vi "DCMotor.vi"(0 "V":dbl, 5 "Omega":dbl, 7 "I":dbl, 9 "dt":dbl, 11 "error in (no error)":errorcluster) -> (4 "Omega Out":dbl, 6 "I Out":dbl, 10 "Torque Out":dbl, 15 "error out":errorcluster)   [LabVIEW 2017]
uses:
  <vilib>/ptbypt/NI_PtbyPt.lvlib
panel:
  in  "Ng":dbl=8.0
  in  "Cs":dbl=0.03
  in  "Cv":dbl=4e-05
  in  "J":dbl=4e-05
  in  "L":dbl=0.8
  in  "R":dbl=7.0
  in  "K":dbl=0.063
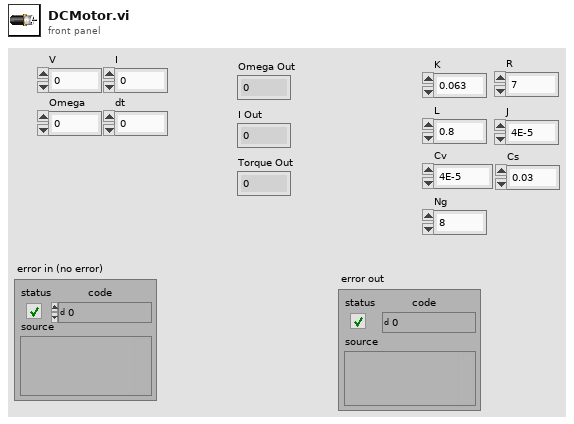
[diagram p1: front panel]
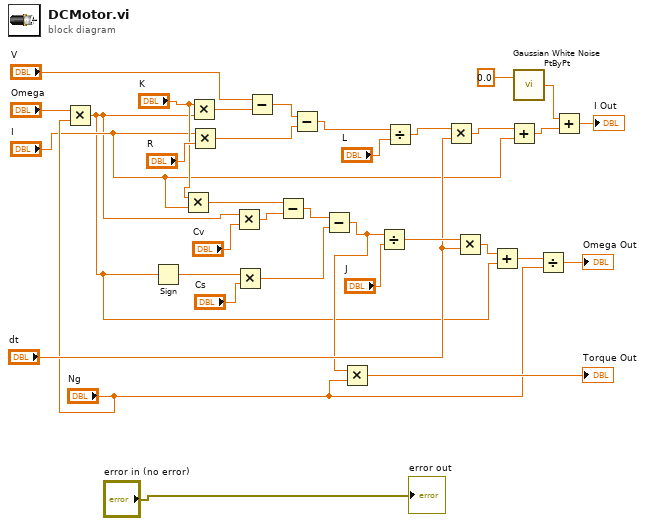
[diagram p0: block diagram]
diagram:
  n1 = Multiply(x="Omega", y="Ng") -> (x*y=w2:dbl)
  n2 = Sign(1:w2) -> (0:w22:dbl)
  n3 = Multiply(x="K", y="I") -> (x*y=w24:dbl)
  n4 = Multiply(x="K", y=w2) -> (x*y=w33:dbl)
  n5 = Multiply(x="I", y="R") -> (x*y=w31:dbl)
  n6 = Multiply(x=w2, y="Cv") -> (x*y=w23:dbl)
  n7 = Multiply(x=w22, y="Cs") -> (x*y=w19:dbl)
  n8 = Subtract(x="V", y=w33) -> (x-y=w32:dbl)
  n9 = Subtract(x=w24, y=w23) -> (x-y=w20:dbl)
  n10 = Subtract(x=w32, y=w31) -> (x-y=w29:dbl)
  n11 = Subtract(x=w20, y=w19) -> (x-y=w14:dbl)
  n12 = Multiply(x=w14, y="Ng") -> (x*y=→"Torque Out":dbl)
  n13 = Divide(x=w14, y="J") -> (x/y=w17:dbl)
  n14 = Divide(x=w29, y="L") -> (x/y=w28:dbl)
  n15 = Multiply(x=w28, y="dt") -> (x*y=w27:dbl)
  n16 = Multiply(x=w17, y="dt") -> (x*y=w15:dbl)
  n17 = Add(x=w15, y=w2) -> (x+y=w11:dbl)
  n18 = Add(x=w27, y="I") -> (x+y=w8:dbl)
  n19 = call <vilib>:"Gaussian White Noise PtByPt.vi"("standard deviation"=0.0 ("amplitude")) -> ("Gaussian white noise"=w6:dbl)  [unwired: 2 in]
  n20 = Divide(x=w11, y="Ng") -> (x/y=→"Omega Out":dbl)
  n21 = Add(x=w6, y=w8) -> (x+y=→"I Out":dbl)
  "error out" <- "error in (no error)"
